vi "Archive Backsave.vi"() -> ()   [LabVIEW 2013, in "LVH-Revert.lvlib"]
uses:
  LVH-Revert.lvlib
  Type Defs/Paths.ctl
  Type Defs/LabVIEW Files.ctl
  <vilib>/LabVIEW Hacker/LVH-Toolbox/Common/Private/Type Defs/LabVIEW Version.ctl
  <vilib>/LabVIEW Hacker/LVH-Toolbox/Common/LVH-Common.lvlib
  Type Defs/Revert Config.ctl
panel:
  in  "Error In":errorcluster
  out "Revert Config":T1={"Revert Paths"={"Archive Path"=path "D:/workspace/revert/todo/todo.zip", "Unzip Directory"=path "D:/workspace/revert/unzip", "Backsave Directory"=path "D:/workspace/revert/backsave", "Output Archive"=path "D:/workspace/revert/output/out.zip", "Backsave Common Directory"=path "D:/workspace/revert/backsave"}, "LabVIEW Files"={"Projects"=[], "Libraries"=[], "Classes"=[], "XControls"=[], "VIs and Controls"=[], "Non LV Files"=[]}, "LabVIEW Version"=enum."8.0"}
  in  "Revert Config":T1={"Revert Paths"={"Archive Path"=path "D:/workspace/revert/todo/todo.zip", "Unzip Directory"=path "D:/workspace/revert/unzip", "Backsave Directory"=path "D:/workspace/revert/backsave", "Output Archive"=path "D:/workspace/revert/output/out.zip", "Backsave Common Directory"=path "D:/workspace/revert/backsave"}, "LabVIEW Files"={"Projects"=[], "Libraries"=[], "Classes"=[], "XControls"=[], "VIs and Controls"=[], "Non LV Files"=[]}, "LabVIEW Version"=enum."8.0"}
  out "Error Out":errorcluster
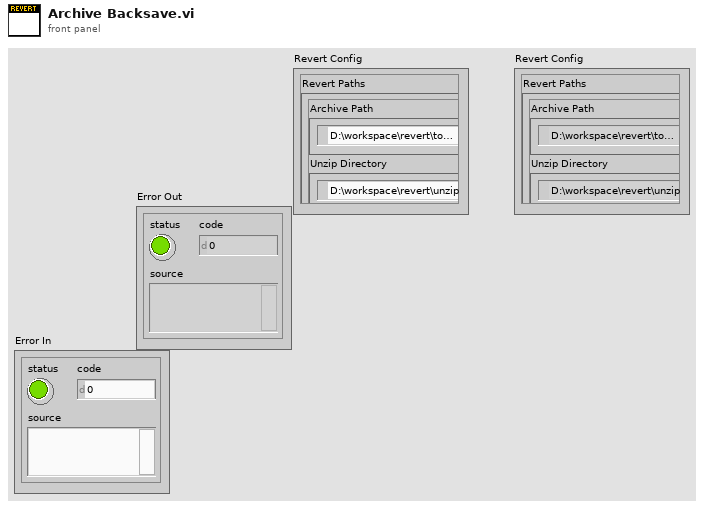
[diagram p1: front panel]
types:
  T1 = typedef "LVH-Revert.lvlib/Revert Config.ctl" = cluster{"Revert Paths":T2, "LabVIEW Files":T3, "LabVIEW Version":T4}
  T2 = typedef "LVH-Revert.lvlib/Paths.ctl" = cluster{"Archive Path":path, "Unzip Directory":path, "Backsave Directory":path, "Output Archive":path, "Backsave Common Directory":path}
  T3 = typedef "LVH-Revert.lvlib/LabVIEW Files.ctl" = cluster{"Projects":path[], "Libraries":path[], "Classes":path[], "XControls":path[], "VIs and Controls":path[], "Non LV Files":path[]}
  T4 = typedef "LVH-Toolbox.lvlib/LVH-Common.lvlib/LabVIEW Version.ctl" = enum16{"8.0", "8.2", "8.6", "9.0", "10.0", "11.0", "12.0", "13.0"}
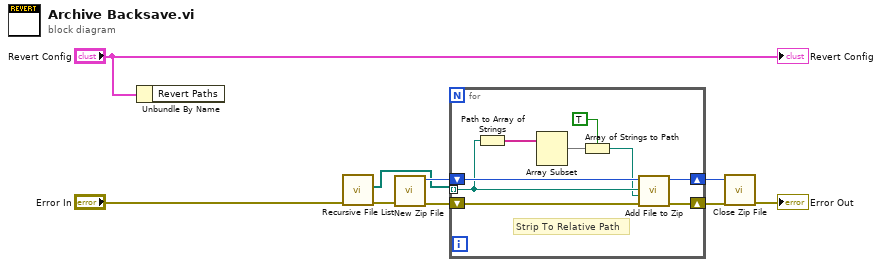
[diagram p0: block diagram]
diagram:
  n1 = Unbundle By Name("Revert Config") -> ()  [unwired: 1 out]
  n2 = call <vilib>:"Recursive File List.vi"("error in (no error)"="Error In") -> ("error out"=w9:errorcluster, "All Files in Dir"=w4:path[])  [unwired: 6 in, 3 out]
  n3 = call <vilib>:"New Zip File.vi"("error in (no error)"=w9) -> ("error out"=w6:errorcluster, "zip file out"=w5:i64)  [unwired: 4 in, 1 out]
  n4 = for {
    tunnel: w4 -> [w11] mode=indexing
    shift-right: [w15] -> w7
    shift-left: w6 -> [w17]
    shift-right: [w16] -> w8
    shift-left: w5 -> [w18]
    # "Strip To Relative Path"
    n5 = Path to Array of Strings(0:w11) -> (2:w14:string[])  [unwired: 1 out]
    n6 = Array Subset(array=w14) -> (w13:string[])  [unwired: 2 in]
    n7 = Array of Strings to Path(0:w13, 1:TRUE ("relative")) -> (2:w10:path)
    n8 = call <vilib>:"Add File to Zip.vi"("error in (no error)"=w17, "destination path in zip"=w10, "source file path"=w11, "zip file in"=w18) -> ("error out"=w15:errorcluster, "zip file out"=w16:i64)  [unwired: 6 in]
  }
  n9 = call <vilib>:"Close Zip File.vi"("error in (no error)"=w7, "zip file in"=w8) -> ("error out"=→"Error Out":errorcluster)  [unwired: 5 in]
  "Revert Config" <- "Revert Config"
